vi "Dictionary to Chart.vi"(8 "error in (no error)":errorcluster, 10 "Display":T1=enum."R and Theta" caption="Enum", 11 "Results (Dictionary)":cluster{"key":string, "value":dbl}[](array[cluster])) -> (0 "error out":errorcluster, 1 "Y/Theta Array":waveform(dbl)[](array[waveform]), 2 "X/R Array":waveform(dbl)[](array[waveform]), 3 "Results (Dictionary) out":cluster{"key":string, "value":dbl}[](array[cluster]))   [LabVIEW 2019, in "Instrument.Lockin.lvlib" / "Instrument UI.Lockin.lvclass"]
uses:
  Instrument UI.Lockin.lvclass
  Typedefs/Display-Enum.ctl
  Instrument.Lockin/Typedefs/Results Type--Enum.ctl
  Instrument.Lockin/Instrument.Lockin.lvclass
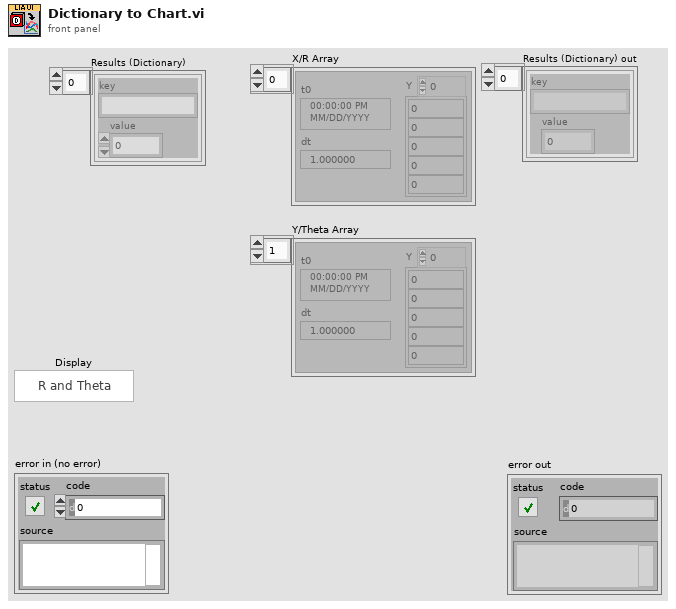
[diagram p1: front panel]
types:
  T1 = typedef "Instrument.Lockin.lvlib/Instrument UI.Lockin.lvclass/Display-Enum.ctl" = enum16{"X and Y", "R and Theta", "Mean"}
  T2 = typedef "Instrument.Lockin.lvlib/Instrument.Lockin.lvclass/Results Type--Enum.ctl" = enum16{"X", "Y", "R", "Theta", "Mean"}
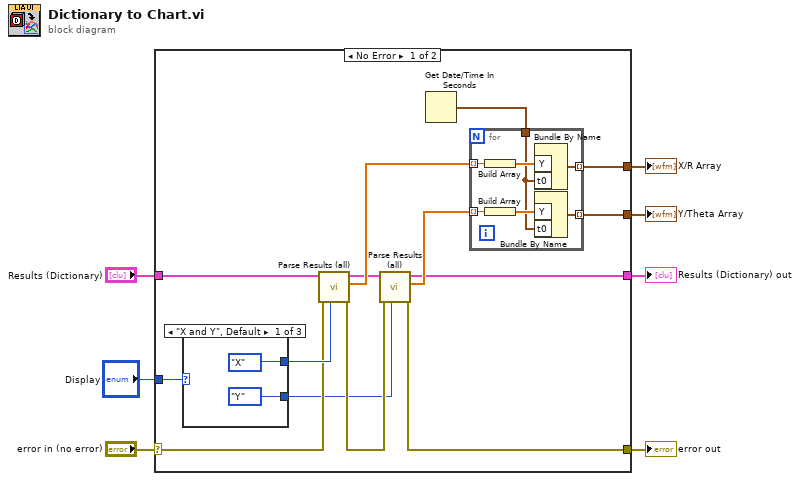
[diagram p0: block diagram]
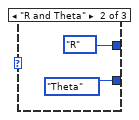
[diagram p2: hidden frame]
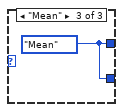
[diagram p3: hidden frame]
diagram:
  n1 = case shown="No Error" "error in (no error)" {
    selector: "error in (no error)" -> [w13 w34]
    tunnel: [w21 _] -> w7
    tunnel: [w20 _] -> w6
    tunnel: "Display" -> [w19 _]
    tunnel: "Results (Dictionary)" -> [w17 _]
    tunnel: [w8 w34] -> w2
    tunnel: [w9 _] -> w1
    frame No Error {
      n2 = case shown="\"X and Y\", Default" w19 {
        tunnel: [Results_Type--Enum."X" ("Type") Results_Type--Enum."R" ("Type") w26] -> w14
        tunnel: [Results_Type--Enum."Y" ("Type") Results_Type--Enum."Theta" ("Type") w26] -> w11
        frame "X and Y", Default {
        }
        frame "R and Theta" {
        }
        frame "Mean" {
          w26 = Results_Type--Enum."Mean" ("Type")
        }
      }
      n3 = call "Parse Results (all).vi"("Type"=w14, "error in (no error)"=w13, "Results (Dictionary)"=w17) -> ("error out"=w12:errorcluster, "Data"=w16:dbl[], "Results (Dictionary)"=w15:cluster{"key":string, "value":dbl}[])  [unwired: 5 in, 1 out]
      n4 = call "Parse Results (all).vi"("Type"=w11, "error in (no error)"=w12, "Results (Dictionary)"=w15) -> ("error out"=w8:errorcluster, "Data"=w10:dbl[], "Results (Dictionary)"=w9:cluster{"key":string, "value":dbl}[])  [unwired: 5 in, 1 out]
      n5 = Get Date/Time In Seconds() -> (seconds since 1Jan1904=w18:timestamp)
      n6 = for {
        tunnel: w16 -> [w33] mode=indexing
        tunnel: w10 -> [w27] mode=indexing
        tunnel: [w32] -> w20 mode=indexing
        tunnel: [w31] -> w21 mode=indexing
        tunnel: w18 -> [w28]
        tunnel: [w27] -> _ mode=indexing
        n7 = Build Array(w33) -> (w30:dbl[])
        n8 = Build Array(w27) -> (w29:dbl[])
        n9 = Bundle By Name("Y"=w30, "t0"=w28) -> (w32:waveform(dbl))  [unwired: 1 in]
        n10 = Bundle By Name("Y"=w29, "t0"=w28) -> (w31:waveform(dbl))  [unwired: 1 in]
      }
    }
    frame Error {
    }
  }
  "Y/Theta Array" <- w7
  "X/R Array" <- w6
  "error out" <- w2
  "Results (Dictionary) out" <- w1
